vi "MeasureRMS.vi"(11 "Digitalizing Parameters":cluster{"Sample Rate":dbl, "# of Cycles":dbl}) -> (7 "Waveform Graph":dynamicdata(graph), 10 "RMS":dbl)   [LabVIEW 2015]
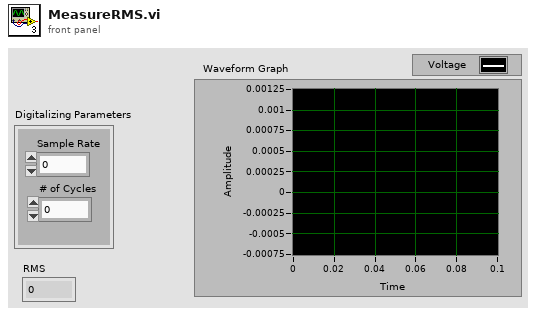
[diagram p1: front panel]
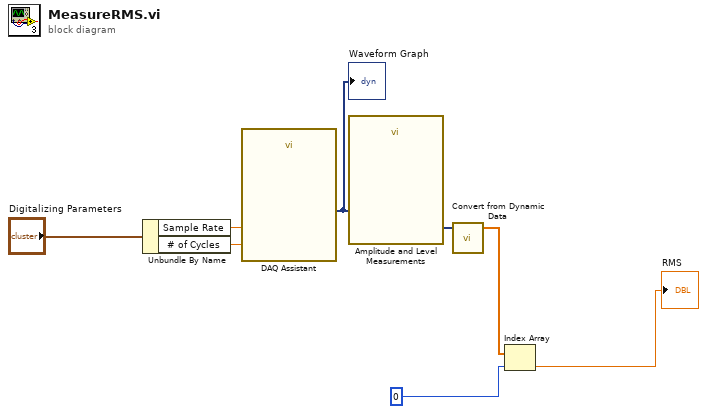
[diagram p0: block diagram]
diagram:
  n1 = Unbundle By Name("Digitalizing Parameters") -> ("Sample Rate"=w7:dbl, "# of Cycles"=w6:dbl)
  n2 = call "DAQ Assistant"("rate"=w7, "number of samples"=w6) -> ("data"=w5:dynamicdata)  [unwired: 15 in, 2 out]
  "Waveform Graph" <- w5
  n3 = call "Amplitude and Level Measurements"("Signals"=w5) -> ("RMS"=w4:dynamicdata)  [unwired: 13 in, 1 out]
  n4 = call "Convert from Dynamic Data"("Dynamic Data Type"=w4) -> ("Array"=w3:dbl[])  [unwired: 3 in]
  n5 = Index Array(array=w3, index=0) -> (element=→"RMS":dbl)
